vi "Main.vi"() -> ()   [LabVIEW 2017]
doc: "The myRIO Project template acquires acceleration data from the onboard accelerometer and displays the changes of acceleration values in a waveform chart."
uses:
  <vilib>/myRIO/Instrument Drivers/Onboard IO/DIO/typedefs/DIO Reference.ctl
  <vilib>/myRIO/Common/Instrument Driver Framework/Utilities/typedefs/myRIO Generic Hardware Reference.ctl
  <vilib>/myRIO/Common/Instrument Driver Framework/Utilities/typedefs/Hardware Version Enum.ctl
  <vilib>/myRIO/Common/Instrument Driver Framework/Utilities/typedefs/myRIO v1.0 Reference.ctl
  <vilib>/myRIO/Common/Instrument Driver Framework/Utilities/typedefs/Generic FPGA Reference.ctl
  <vilib>/myRIO/Common/Instrument Driver Framework/myRIO v1.0/DIO/typedefs/DIO Channels List.ctl
  <vilib>/myRIO/Common/Instrument Driver Framework/myRIO v1.0/DIO/typedefs/DIO Channels Enum.ctl
  <vilib>/userdefined/High Color/nirio_resource_hc.ctl
  <vilib>/myRIO/Instrument Drivers/Onboard IO/AI/typedefs/AI Reference.ctl
  <vilib>/myRIO/Common/Instrument Driver Framework/myRIO v1.0/AI/typedefs/AI Channels List.ctl
  <vilib>/myRIO/Common/Instrument Driver Framework/myRIO v1.0/AI/typedefs/AI Channels Enum.ctl
  <vilib>/myRIO/Common/Instrument Driver Framework/Utilities/typedefs/Analog Scaling Constants List.ctl
  <vilib>/myRIO/Common/Instrument Driver Framework/Utilities/typedefs/Analog Scaling Constants.ctl
  <vilib>/myRIO/Instrument Drivers/Onboard Devices/Accelerometer/typedefs/Accelerometer Reference.ctl
  <vilib>/myRIO/Common/Instrument Driver Framework/myRIO v1.0/Accelerometer/typedefs/Accelerometer Channels List.ctl
  <vilib>/myRIO/Common/Instrument Driver Framework/myRIO v1.0/Accelerometer/typedefs/Accelerometer Channels Enum.ctl
  <vilib>/myRIO/Instrument Drivers/Onboard IO/PWM/typedefs/PWM Reference.ctl
  <vilib>/myRIO/Common/Instrument Driver Framework/myRIO v1.0/PWM/typedefs/PWM Channels Enum.ctl
  <vilib>/myRIO/Instrument Drivers/Onboard IO/PWM/typedefs/PWM Configuration.ctl
  <vilib>/myRIO/Common/Instrument Driver Framework/Utilities/vis/Is FPGA Ref Available.vi
  <vilib>/myRIO/Common/Instrument Driver Framework/myRIO v1.0/DIO/vis/myRIO v1.1 Open DIO.vi
  <vilib>/myRIO/Instrument Drivers/Onboard IO/DIO/vis/Write.vi
  <vilib>/myRIO/Instrument Drivers/Onboard IO/DIO/vis/Read.vi
  <vilib>/myRIO/Common/Instrument Driver Framework/myRIO v1.0/PWM/vis/myRIO v1.1 Open PWM.vi
  <vilib>/myRIO/Instrument Drivers/Onboard IO/PWM/vis/Set Duty Cycle and Frequency.vi
  <vilib>/myRIO/Common/Instrument Driver Framework/myRIO v1.0/Accelerometer/vis/myRIO v1.1 Open Accelerometer.vi
  <vilib>/myRIO/Instrument Drivers/Onboard Devices/Accelerometer/vis/Read.vi
  <vilib>/myRIO/Common/Instrument Driver Framework/myRIO v1.0/AI/vis/myRIO v1.1 Open AI.vi
  <vilib>/myRIO/Instrument Drivers/Onboard IO/AI/vis/Read.vi
  <vilib>/myRIO/Common/Instrument Driver Framework/Utilities/vis/Validate Channels.vi
  <vilib>/myRIO/Common/Instrument Driver Framework/myRIO v1.0/DIO/vis/myRIO v1.0 Reserve DIO.vi
  <vilib>/myRIO/Common/Instrument Driver Framework/myRIO v1.0/PWM/vis/myRIO v1.0 Reserve PWM.vi
  <vilib>/myRIO/Common/Instrument Driver Framework/myRIO v1.0/Accelerometer/vis/myRIO v1.0 Reserve Accelerometer.vi
  <vilib>/myRIO/Common/Instrument Driver Framework/myRIO v1.0/AI/vis/myRIO v1.0 Reserve AI.vi
  <vilib>/myRIO/Common/Instrument Driver Framework/myRIO v1.0/UART/vis/myRIO v1.0 Close UART.vi
  <vilib>/myRIO/Common/Instrument Driver Framework/myRIO v1.0/Resource Manager/vis/myRIO v1.0 Reserve Channel List.vi
  <vilib>/myRIO/Common/Instrument Driver Framework/myRIO v1.0/DIO/vis/myRIO v1.0 Build MUX Configuration DIO.vi
  <vilib>/myRIO/Common/Instrument Driver Framework/myRIO v1.0/PWM/vis/myRIO v1.0 Build MUX Configuration PWM.vi
  <vilib>/myRIO/Common/Instrument Driver Framework/myRIO v1.0/Accelerometer/vis/myRIO v1.0 Build MUX Configuration Accelerometer.vi
  <vilib>/myRIO/Common/Instrument Driver Framework/myRIO v1.0/AI/vis/myRIO v1.0 Build MUX Configuration AI.vi
  <vilib>/myRIO/Common/Instrument Driver Framework/myRIO v1.0/Resource Manager/vis/myRIO v1.0 Reserve Channel.vi
  <vilib>/myRIO/Common/Instrument Driver Framework/myRIO v1.0/Resource Manager/vis/myRIO v1.0 Unreserve Channel.vi
  <vilib>/myRIO/Common/Instrument Driver Framework/myRIO v1.0/Resource Manager/vis/myRIO v1.0 Create Configuration List.vi
  <vilib>/myRIO/Common/Instrument Driver Framework/myRIO v1.0/Resource Manager/vis/myRIO v1.0 Build Mutex Name.vi
  <vilib>/Utility/VariantDataType/GetNumericInfo.vi
  <vilib>/Utility/error.llb/Error Cluster From Error Code.vi
  <vilib>/myRIO/Common/Instrument Driver Framework/myRIO v1.0/myRIO v1.1 Open.vi
  <vilib>/myRIO/Common/Instrument Driver Framework/Utilities/vis/IO Manager.vi
  <vilib>/myRIO/Common/Instrument Driver Framework/Utilities/vis/Configuration Manager.vi
  <vilib>/myRIO/Common/Instrument Driver Framework/myRIO v1.0/Resource Manager/vis/myRIO v1.0 Configure IO.vi
  <vilib>/myRIO/Common/Instrument Driver Framework/myRIO v1.0/myRIO v1.0 Close.vi
  <vilib>/myRIO/Common/Instrument Driver Framework/myRIO v1.0/DIO/vis/myRIO v1.0 Write DIO.vi
  <vilib>/myRIO/Common/Instrument Driver Framework/myRIO v1.0/AI/vis/myRIO v1.0 Get Scaling Constants AI.vi
  <vilib>/myRIO/Common/Instrument Driver Framework/myRIO v1.0/AI/vis/myRIO v1.0 Read AI.vi
  <vilib>/myRIO/Common/Instrument Driver Framework/myRIO v1.0/Accelerometer/vis/myRIO v1.0 Get Scaling Constant Accelerometer.vi
  <vilib>/myRIO/Common/Instrument Driver Framework/myRIO v1.0/Accelerometer/vis/myRIO v1.0 Read Accelerometer.vi
  <vilib>/myRIO/Common/Instrument Driver Framework/myRIO v1.0/DIO/vis/myRIO v1.0 Read DIO.vi
  <vilib>/myRIO/Common/Instrument Driver Framework/myRIO v1.0/PWM/vis/myRIO v1.0 Write PWM.vi
  <vilib>/myRIO/Common/Instrument Driver Framework/Utilities/vis/FPGA Ref Manager.vi
  <vilib>/myRIO/Common/Instrument Driver Framework/myRIO v1.0/myRIO v1.0 Reset FPGA.vi
  <vilib>/myRIO/Common/Instrument Driver Framework/myRIO v1.0/IRQ/vis/myRIO v1.0 IRQ Info FGV.vi
  <vilib>/myRIO/Common/Instrument Driver Framework/myRIO v1.0/IRQ/vis/myRIO v1.0 Timer IRQ Info FGV.vi
  <vilib>/myRIO/Common/Instrument Driver Framework/myRIO v1.0/IRQ/vis/myRIO v1.0 ISR Agent.vi
  <vilib>/myRIO/Express VI/Onboard Devices/LED/LED Express VI.xnode
  <vilib>/myRIO/Instrument Drivers/Onboard IO/DIO/vis/myRIO DIO Open.xnode
  <vilib>/myRIO/Express VI/Onboard IO/AI/AI Express VI.xnode
  <vilib>/myRIO/Instrument Drivers/Onboard IO/AI/vis/myRIO AI Open.xnode
  <vilib>/myRIO/Express VI/Onboard Devices/Accelerometer/Accelerometer Express VI.xnode
  <vilib>/myRIO/Instrument Drivers/Onboard Devices/Accelerometer/vis/myRIO Accelerometer Open.xnode
  <vilib>/myRIO/Express VI/Onboard Devices/Button/Button Express VI.xnode
  <vilib>/myRIO/Express VI/Onboard IO/PWM/PWM Express VI.xnode
  <vilib>/myRIO/Instrument Drivers/Onboard IO/PWM/vis/myRIO PWM Open.xnode
  <vilib>/myRIO/Instrument Drivers/Utilities/Utilities.lvlib
  <vilib>/myRIO/Instrument Drivers/Onboard IO/AI/AI.lvlib
  <vilib>/myRIO/Instrument Drivers/Onboard IO/PWM/PWM.lvlib
  <vilib>/myRIO/Instrument Drivers/Onboard IO/DIO/DIO.lvlib
  <vilib>/myRIO/Instrument Drivers/Onboard Devices/Accelerometer/Accelerometer.lvlib
panel:
  out "Valve Open":bool
  out "TCP Listen":bool
  out "Reset":bool
  out "Z-Axis":dbl
  out "Y-Axis":dbl
  out "X-Axis":dbl
  out "Accelerometer":cluster{dbl, dbl, dbl}(graph)
  out "Temperature\nMeter":dbl(knob) scale=0.0..100.0
  in  "Max Temperature":dbl
  in  "Front Controller Password":dbl
  in  "STOP SYSTEM":bool
  in  "Max Movement":dbl min=1.0
  out "Self-destruct Timer":i32
  out "Mode":string
  out "Self-destruct Cancelled":bool
  out "Local Cooling Request":bool
  out "Self-destructed":bool
  out "Self-destruct Timer":bool
  out "Movement Detected":bool
  out "Instructions":string
  out "Message Number":dbl
  out "Received Cluster":T1
  out "Front Controller":bool
  out "Local":bool
  out "Bytes written":i32
  out "Send Cluster":T2
  # "LED Indicators"
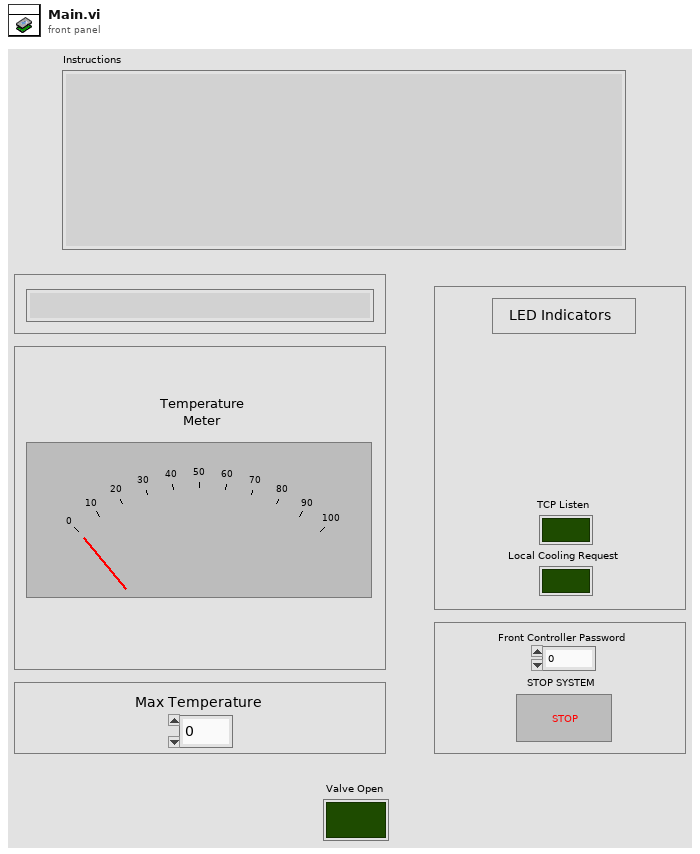
[diagram p1: front panel]
types:
  T1 = cluster{"Servo Open":bool, "Self-Destruct":bool, "Front Controller Passcode":dbl}
  T2 = cluster{"Temperature":dbl, "X - Axis":dbl, "Y - Axis":dbl, "Z - Axis":dbl, "Movement":bool, "Message":dbl, "LCR":bool, "Numeric":dbl}
  T3 = typedef "DIO.lvlib/DIO Reference.ctl" = cluster{"myRIO Reference":T4, "DIO Channels List":T8}
  T4 = typedef "myRIO Generic Hardware Reference.ctl" = cluster{"myRIO Model":T5, "myRIO Hardware Reference":T6}
  T5 = typedef "Hardware Version Enum.ctl" = enum16{"Unknown", "myRIO-1900", "myRIO-1950", "roboRIO", "NI ELVIS RIO CM"}
  T6 = typedef "myRIO v1.0 Reference.ctl" = cluster{"Generic FPGA Reference":T7, "Allow multiple opens":bool}
  T7 = typedef "Generic FPGA Reference.ctl" = refnum<k20>
  T8 = typedef "DIO Channels List.ctl" = T9[]
  T9 = typedef "DIO Channels Enum.ctl" = enum16{"Not Connected", "C/DIO0", "C/DIO1", "C/DIO2", "C/DIO3", "C/DIO4", "C/DIO5", "C/DIO6", "C/DIO7", "A/DIO0", "A/DIO1", "A/DIO2", "A/DIO3", "A/DIO4", "A/DIO5", "A/DIO6", "A/DIO7", "A/DIO8", "A/DIO9", "A/DIO10", "A/DIO11", "A/DIO12", "A/DIO13", "A/DIO14", "A/DIO15", "B/DIO0", "B/DIO1", "B/DIO2", "B/DIO3", "B/DIO4", "B/DIO5", "B/DIO6", "B/DIO7", "B/DIO8", "B/DIO9", "B/DIO10", "B/DIO11", "B/DIO12", "B/DIO13", "B/DIO14", "B/DIO15", "LED0", "LED1", "LED2", "LED3", "Button0", "DIO/DIO0", "DIO/DIO1", "DIO/DIO2", "DIO/DIO3", "DIO/DIO4", "DIO/DIO5", "DIO/DIO6", "DIO/DIO7", "DIO/DIO8", "DIO/DIO9", "SPI/CS0", "SPI/CS1", "SPI/CS2", "SPI/CS3", "LED RADIO (Green)", "LED RADIO (Red)", "LED COMM (Green)", "LED COMM (Red)", "LED MODE (Green)", "LED MODE (Red)"}
  T10 = typedef "nirio_resource_hc.ctl" = tag
  T11 = typedef "PWM.lvlib/PWM Reference.ctl" = cluster{"myRIO Reference":T4, "PWM Channels Enum":T12, "PWM Configuration":T13}
  T12 = typedef "PWM Channels Enum.ctl" = enum16{"Not Connected", "C/PWM0", "C/PWM1", "A/PWM0", "A/PWM1", "A/PWM2", "B/PWM0", "B/PWM1", "B/PWM2", "PWM/PWM0", "PWM/PWM1", "PWM/PWM2", "PWM/PWM3", "PWM/PWM4", "PWM/PWM5", "PWM/PWM6", "PWM/PWM7", "PWM/PWM8", "PWM/PWM9"}
  T13 = typedef "PWM.lvlib/PWM Configuration.ctl" = cluster{"Frequency":dbl, "Duty Cycle":dbl}
  T14 = typedef "Accelerometer.lvlib/Accelerometer Reference.ctl" = cluster{"myRIO Reference":T4, "Accelerometer Channels List":T15, "LSB Weight":dbl}
  T15 = typedef "Accelerometer Channels List.ctl" = T16[]
  T16 = typedef "Accelerometer Channels Enum.ctl" = enum16{"Not Connected", "X-Axis", "Y-Axis", "Z-Axis"}
  T17 = typedef "AI.lvlib/AI Reference.ctl" = cluster{"myRIO Reference":T4, "AI Channels List":T18, "AI Scaling Constants List":T20}
  T18 = typedef "AI Channels List.ctl" = T19[]
  T19 = typedef "AI Channels Enum.ctl" = enum16{"Not Connected", "AudioIn/Left", "AudioIn/Right", "C/AI0", "C/AI1", "A/AI0", "A/AI1", "A/AI2", "A/AI3", "B/AI0", "B/AI1", "B/AI2", "B/AI3", "AI/AI0", "AI/AI1", "AI/AI2", "AI/AI3"}
  T20 = typedef "Analog Scaling Constants List.ctl" = T21[]
  T21 = typedef "Analog Scaling Constants.ctl" = cluster{"LSB Weight (Volts)":dbl, "Offset (Volts)":dbl, "Signed?":bool}
  T22 = cluster{dbl, "X-Axis":dbl, "Y-Axis":dbl, dbl, "Movement Detected":bool, "Message Number":dbl, "Local Cooling Request":bool, "Front Controller Password":dbl}
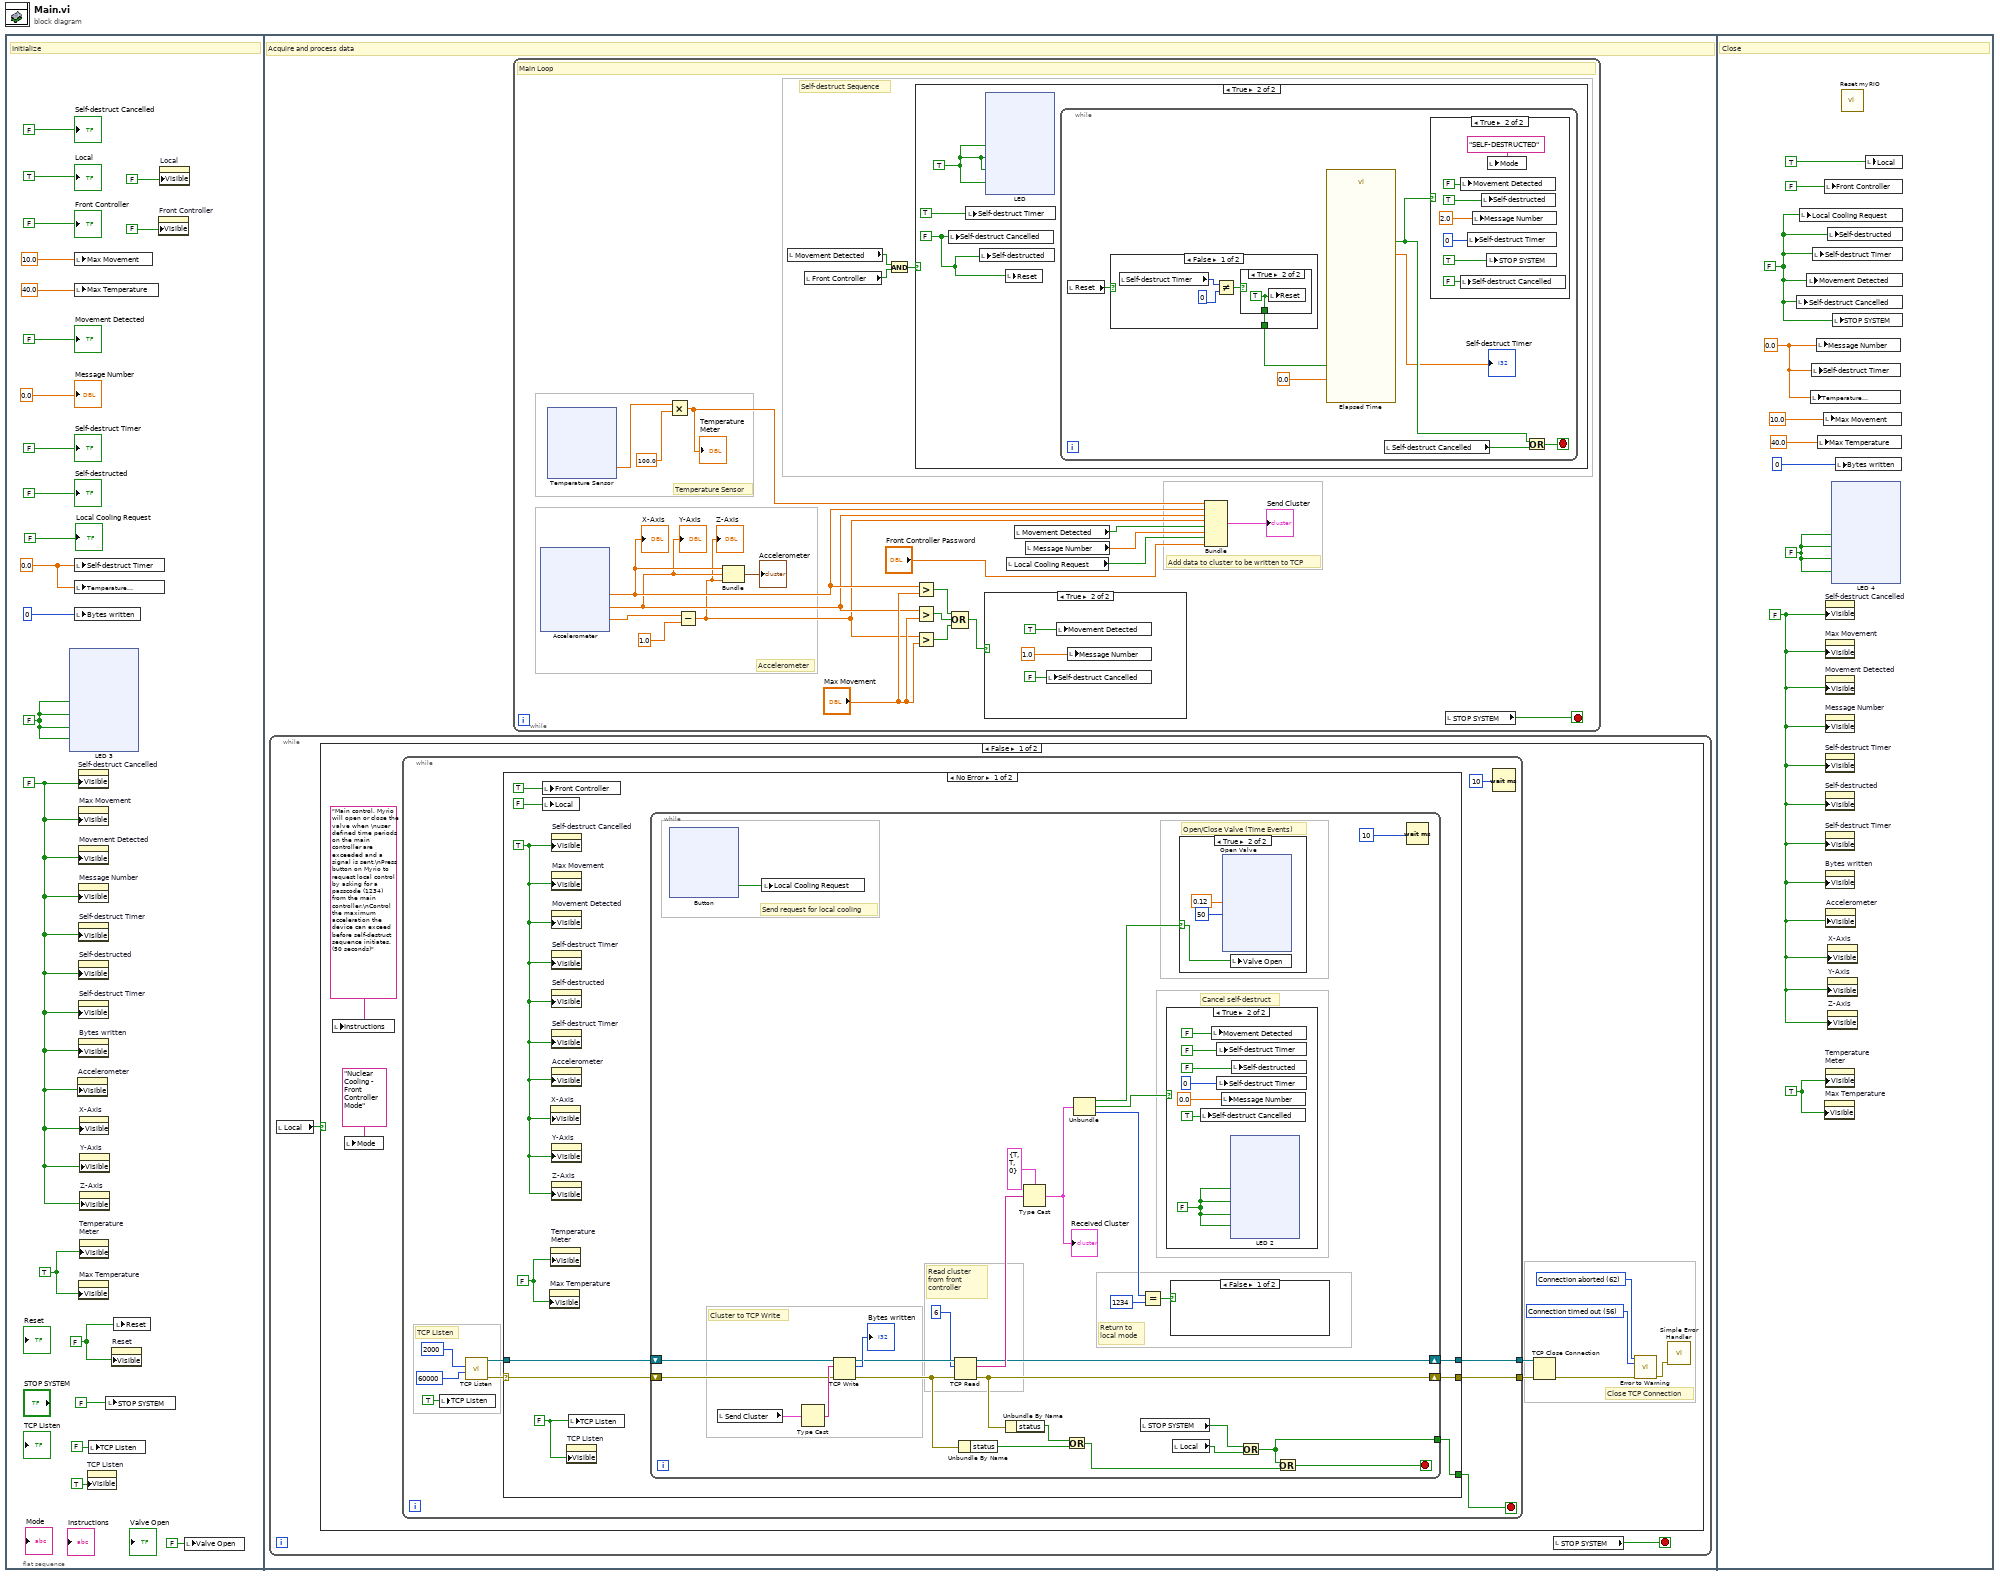
[diagram p0: block diagram]
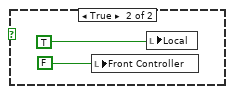
[diagram p2: hidden frame]
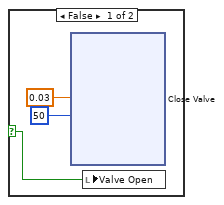
[diagram p4: hidden frame]
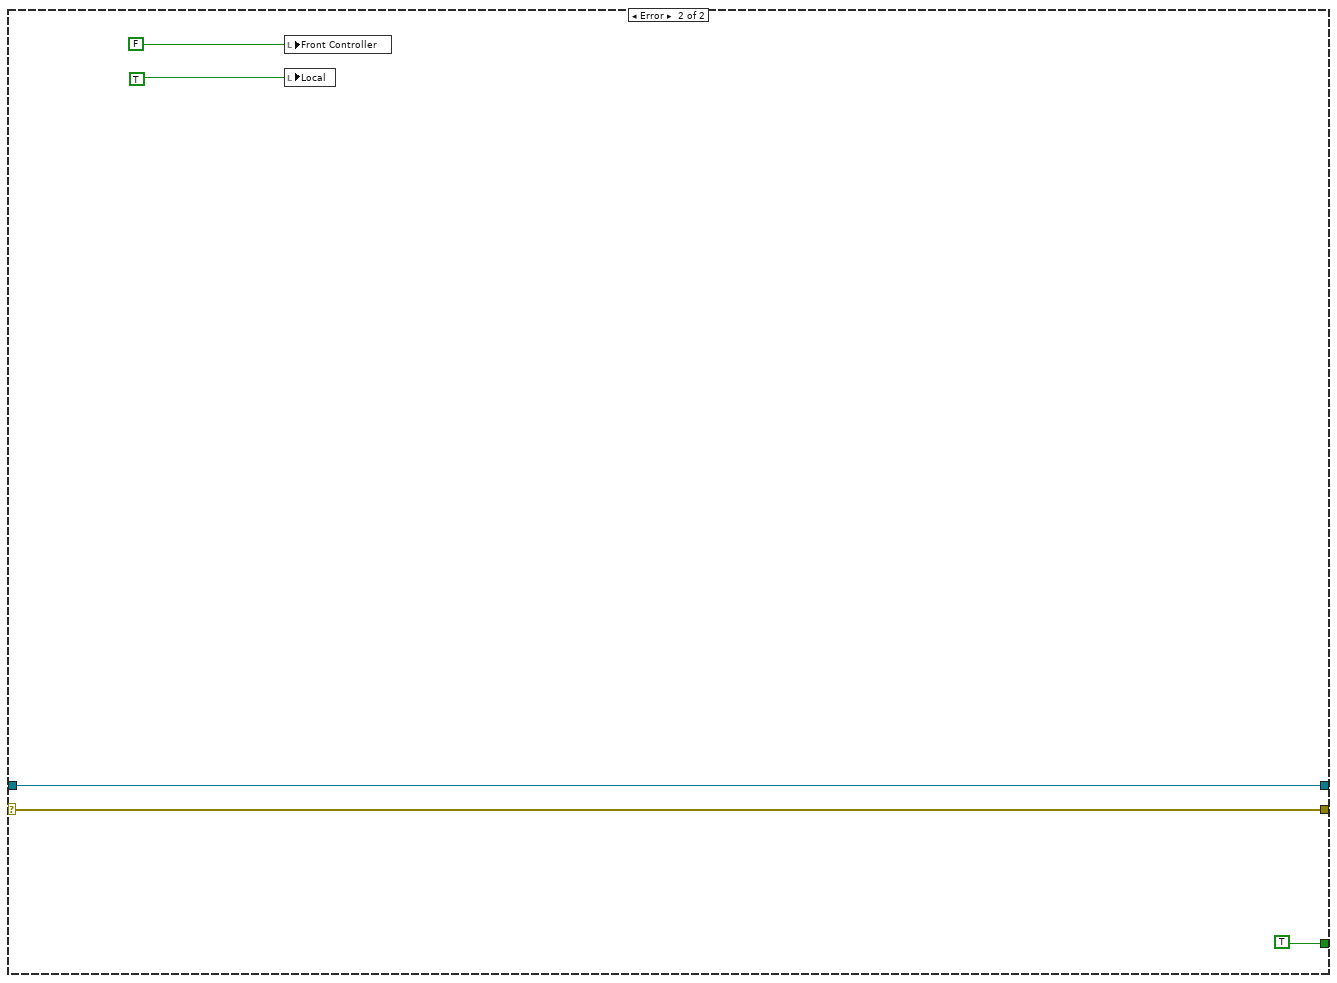
[diagram p5: hidden frame]
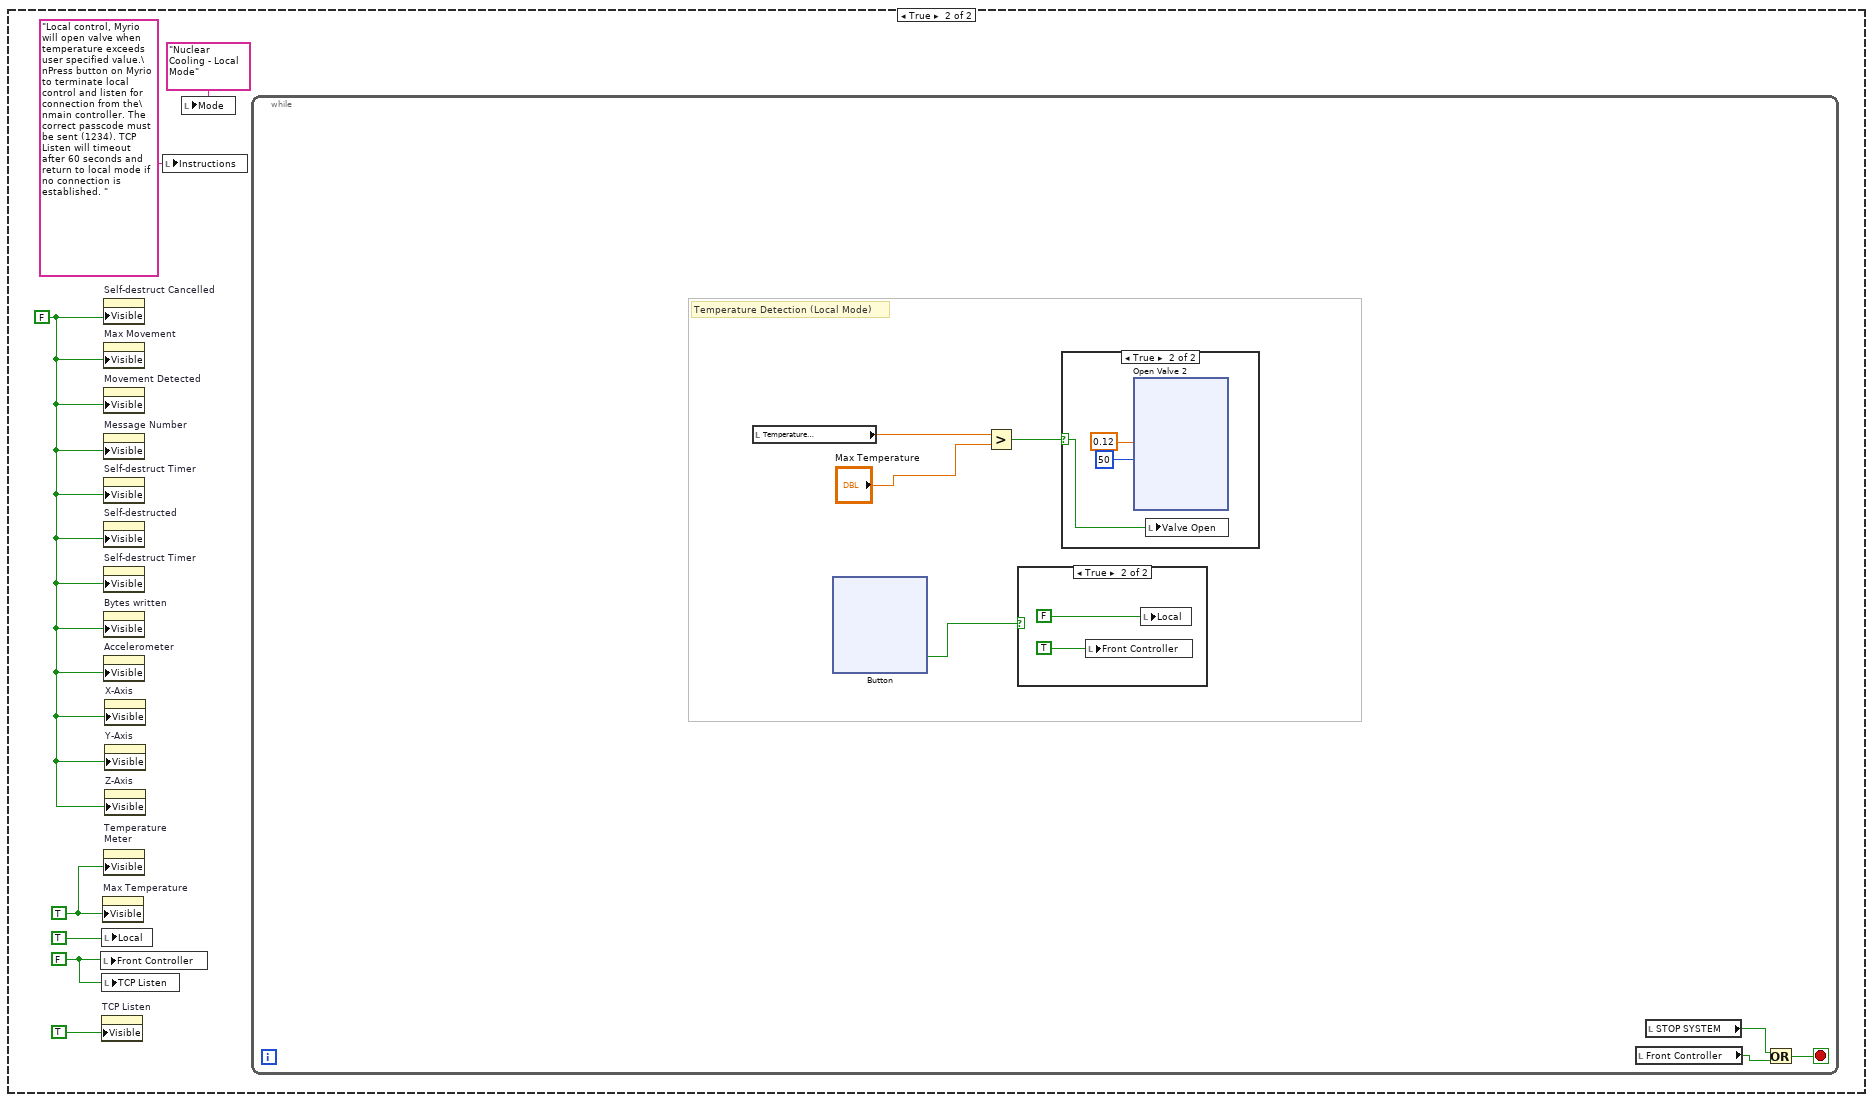
[diagram p6: hidden frame]
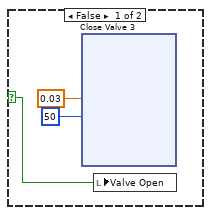
[diagram p8: hidden frame]
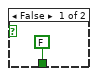
[diagram p10: hidden frame]
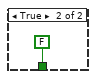
[diagram p11: hidden frame]
diagram:
  n1 = flat-sequence {
    frame #0 {
      w2 = FALSE
      w6 = TRUE
      w5 = FALSE
      w15 = FALSE
      w7 = 0.0
      # "Initialize"
      n2 = xnode "LED 3"("LED0"=w15, "LED1"=w15, "LED2"=w15, "LED3"=w15) -> ()  [unwired: 1 in, 1 out]
      n3 = local write "Max Movement"(10.0) -> ()
      n4 = local write "Max Temperature"(40.0) -> ()
      n5 = local write "Self-destruct Timer"(w7) -> ()
      n6 = local write "Temperature\nMeter"(w7) -> ()
      n7 = local write "Bytes written"(0) -> ()
      n8 = property on="Accelerometer" class="WFChart (strict)"("Visible"=w5) -> ()  [unwired: 2 in, 2 out]
      n9 = property on="Self-destruct Cancelled" class="Bool (strict)"("Visible"=w5) -> ()  [unwired: 2 in, 2 out]
      n10 = property on="Max Movement" class="DigNum (strict)"("Visible"=w5) -> ()  [unwired: 2 in, 2 out]
      n11 = property on="Movement Detected" class="Bool (strict)"("Visible"=w5) -> ()  [unwired: 2 in, 2 out]
      n12 = property on="Message Number" class="DigNum (strict)"("Visible"=w5) -> ()  [unwired: 2 in, 2 out]
      n13 = property on="Self-destruct Timer" class="Bool (strict)"("Visible"=w5) -> ()  [unwired: 2 in, 2 out]
      n14 = property on="Self-destructed" class="Bool (strict)"("Visible"=w5) -> ()  [unwired: 2 in, 2 out]
      n15 = property on="Self-destruct Timer" class="DigNum (strict)"("Visible"=w5) -> ()  [unwired: 2 in, 2 out]
      n16 = property on="Bytes written" class="DigNum (strict)"("Visible"=w5) -> ()  [unwired: 2 in, 2 out]
      n17 = property on="Max Temperature" class="DigNum (strict)"("Visible"=w6) -> ()  [unwired: 2 in, 2 out]
      n18 = property on="X-Axis" class="DigNum (strict)"("Visible"=w5) -> ()  [unwired: 2 in, 2 out]
      n19 = property on="Temperature\nMeter" class="Knob (strict)"("Visible"=w6) -> ()  [unwired: 2 in, 2 out]
      n20 = property on="Y-Axis" class="DigNum (strict)"("Visible"=w5) -> ()  [unwired: 2 in, 2 out]
      n21 = property on="Z-Axis" class="DigNum (strict)"("Visible"=w5) -> ()  [unwired: 2 in, 2 out]
      n22 = property on="TCP Listen" class="Bool (strict)"("Visible"=TRUE) -> ()  [unwired: 2 in, 2 out]
      n23 = local write "TCP Listen"(FALSE) -> ()
      n24 = local write "STOP SYSTEM"(FALSE) -> ()
      n25 = property on="Reset" class="Bool (strict)"("Visible"=w2) -> ()  [unwired: 2 in, 2 out]
      n26 = local write "Reset"(w2) -> ()
      n27 = property on="Front Controller" class="Bool (strict)"("Visible"=FALSE) -> ()  [unwired: 2 in, 2 out]
      n28 = property on="Local" class="Bool (strict)"("Visible"=FALSE) -> ()  [unwired: 2 in, 2 out]
      n29 = local write "Valve Open"(FALSE) -> ()
      "Local" <- TRUE
      "Front Controller" <- FALSE
      "Movement Detected" <- FALSE
      "Message Number" <- 0.0
      "Self-destruct Timer" <- FALSE
      "Self-destruct Cancelled" <- FALSE
      "Self-destructed" <- FALSE
      "Local Cooling Request" <- FALSE
    }
    frame #1 {
      # "Acquire and process data"
      n30 = while {
        stop <- w61 stop-if-true
        n31 = local read "Local"() -> (w62:bool)
        n32 = case shown="False" w62 {
          frame False {
            w66 = 56 items=["No Error", "Argument Error", "Memory Full", "Out of Zone", "End of File", "File Already Open", "Generic File IO Error", "File Not Found", "File Permission Error", "Disk Full", "Duplicate Path", "Too Many Files Open", "Not Enabled", "Resource File Not Found", "Cannot Add Resource", "Resource Not Found", "Image Not Found", "Image Memory Error", "Pen Does Not Exist", "Config Bad Type", "Config Token Not Found", "Config Parse Error", "Config Memory Error", "Bad External Code Format", "Bad External Code Offset", "External Code Not Present", "Null Window", "Destroy Window Mixup", "Null Menu", "Print Aborted", "Bad Print Record", "Print Driver Error", "Windows Error During Print", "Memory Error During Print", "Print Dialog Error", "Generic Print Error", "Invalid Device Refnum", "Device Not Found", "Device Parameter Error", "Device Unit Error", "Can't Open Device", "Device Call Aborted", "Generic Error", "Cancelled By User", "Object ID Too Low", "Object ID Too High", "Object Not In Heap", "Unknown Heap", "Bad DefProc ID", "DefProc Not In Table", "Message Out Of Range", "Null Method", "Unknown Message", "Manager Call Not Supported", "Bad address", "Connection In progress", "Connection timed out", "Connection is already in progress", "Network attribute not supported", "Network error", "Address in use", "System out of memory", "Connection aborted", "Connection refused", "Connection is not connected", "Connection is already connected", "Connection closed", "Initialize error (interapplication manager)", "Bad occurrence", "Wait on unbound occurrence handler", "Occurrence queue overflow", "Bad path", "Semaphore not signaled", "Unrecognized type (interapplication manager)"] ("3rd Error to Convert")
            w67 = 62 items=["No Error", "Argument Error", "Memory Full", "Out of Zone", "End of File", "File Already Open", "Generic File IO Error", "File Not Found", "File Permission Error", "Disk Full", "Duplicate Path", "Too Many Files Open", "Not Enabled", "Resource File Not Found", "Cannot Add Resource", "Resource Not Found", "Image Not Found", "Image Memory Error", "Pen Does Not Exist", "Config Bad Type", "Config Token Not Found", "Config Parse Error", "Config Memory Error", "Bad External Code Format", "Bad External Code Offset", "External Code Not Present", "Null Window", "Destroy Window Mixup", "Null Menu", "Print Aborted", "Bad Print Record", "Print Driver Error", "Windows Error During Print", "Memory Error During Print", "Print Dialog Error", "Generic Print Error", "Invalid Device Refnum", "Device Not Found", "Device Parameter Error", "Device Unit Error", "Can't Open Device", "Device Call Aborted", "Generic Error", "Cancelled By User", "Object ID Too Low", "Object ID Too High", "Object Not In Heap", "Unknown Heap", "Bad DefProc ID", "DefProc Not In Table", "Message Out Of Range", "Null Method", "Unknown Message", "Manager Call Not Supported", "Bad address", "Connection In progress", "Connection timed out", "Connection is already in progress", "Network attribute not supported", "Network error", "Address in use", "System out of memory", "Connection aborted", "Connection refused", "Connection is not connected", "Connection is already connected", "Connection closed", "Initialize error (interapplication manager)", "Bad occurrence", "Wait on unbound occurrence handler", "Occurrence queue overflow", "Bad path", "Semaphore not signaled", "Unrecognized type (interapplication manager)"] ("1st Error to Convert")
            # "Close TCP Connection"
            n33 = local write "Instructions"("Main control, Myrio will open or close the valve when \nuser defined time periods on the main controller are exceeded and a signal is sent.\nPress button on Myrio to request local control by asking for a passcode (1234) from the main controller.\nControl the maximum acceleration the device can exceed before self-destruct sequence initiates. (50 seconds)") -> ()
            n34 = local write "Mode"("Nuclear Cooling - Front Controller Mode") -> ()
            n35 = while {
              tunnel: [w73] -> w69
              tunnel: [w72] -> w68
              stop <- w76 stop-if-true
              # "TCP Listen"
              n36 = local write "TCP Listen"(TRUE) -> ()
              n37 = call <vilib>:"TCP Listen.vi"("timeout ms (wait forever: -1)"=60000, "port"=u16 2000 ("timeout ms (wait forever: -1)")) -> ("error out"=w75:errorcluster, "connection ID"=w74:refnum<k5>)  [unwired: 2 in, 6 out]
              n38 = case shown="No Error" w75 {
                selector: w75 -> [w89 w278]
                tunnel: [w88 TRUE] -> w76
                tunnel: w74 -> [w87 w279]
                tunnel: [w86 w279] -> w73
                tunnel: [w85 w278] -> w72
                frame No Error {
                  w80 = FALSE
                  w82 = FALSE
                  w81 = TRUE
                  n39 = local write "Front Controller"(TRUE) -> ()
                  n40 = local write "Local"(FALSE) -> ()
                  n41 = property on="Max Temperature" class="DigNum (strict)"("Visible"=w82) -> ()  [unwired: 2 in, 2 out]
                  n42 = property on="X-Axis" class="DigNum (strict)"("Visible"=w81) -> ()  [unwired: 2 in, 2 out]
                  n43 = property on="Temperature\nMeter" class="Knob (strict)"("Visible"=w82) -> ()  [unwired: 2 in, 2 out]
                  n44 = property on="Self-destruct Cancelled" class="Bool (strict)"("Visible"=w81) -> ()  [unwired: 2 in, 2 out]
                  n45 = property on="Max Movement" class="DigNum (strict)"("Visible"=w81) -> ()  [unwired: 2 in, 2 out]
                  n46 = property on="Movement Detected" class="Bool (strict)"("Visible"=w81) -> ()  [unwired: 2 in, 2 out]
                  n47 = property on="Self-destruct Timer" class="Bool (strict)"("Visible"=w81) -> ()  [unwired: 2 in, 2 out]
                  n48 = property on="Self-destructed" class="Bool (strict)"("Visible"=w81) -> ()  [unwired: 2 in, 2 out]
                  n49 = property on="Self-destruct Timer" class="DigNum (strict)"("Visible"=w81) -> ()  [unwired: 2 in, 2 out]
                  n50 = property on="Accelerometer" class="WFChart (strict)"("Visible"=w81) -> ()  [unwired: 2 in, 2 out]
                  n51 = property on="Y-Axis" class="DigNum (strict)"("Visible"=w81) -> ()  [unwired: 2 in, 2 out]
                  n52 = property on="Z-Axis" class="DigNum (strict)"("Visible"=w81) -> ()  [unwired: 2 in, 2 out]
                  n53 = property on="TCP Listen" class="Bool (strict)"("Visible"=w80) -> ()  [unwired: 2 in, 2 out]
                  n54 = local write "TCP Listen"(w80) -> ()
                  n55 = while {
                    shift-right: [w103] -> w86
                    shift-left: w87 -> [w112]
                    shift-right: [w102] -> w85
                    shift-left: w89 -> [w114]
                    tunnel: [w90] -> w88
                    stop <- w104 stop-if-true
                    # "Return to \nlocal mode"
                    # "Cancel self-destruct"
                    # "Open/Close Valve (Time Events)"
                    # "Read cluster \nfrom front controller"
                    # "Send request for local cooling"
                    # "Cluster to TCP Write"
                    n56 = xnode "Button"() -> ("Value"=w96:bool)  [unwired: 1 in, 1 out]
                    n57 = local read "Send Cluster"() -> (w113:T2)
                    n58 = local write "Local Cooling Request"(w96) -> ()
                    n59 = Type Cast(x=w113) -> (*(type *) &x=w116:string)  [unwired: 1 out]
                    n60 = TCP Write(connection ID=w112, data in=w116, error in (no error)=w114) -> (connection ID out=w111:refnum<k5>, bytes written=→"Bytes written":i32, error out=w108:errorcluster)  [unwired: 1 out]
                    n61 = TCP Read(connection ID=w111, bytes to read=6, error in (no error)=w108) -> (connection ID out=w103:refnum<k5>, data out=w109:string, error out=w102:errorcluster)  [unwired: 2 in]
                    n62 = Unbundle By Name(w108) -> ("status"=w107:bool)
                    n63 = Unbundle By Name(w102) -> ("status"=w106:bool)
                    n64 = Type Cast(type=cluster{bool, bool, i32} {TRUE, TRUE, 0}, x=w109) -> (*(type *) &x=w100:cluster{bool, bool, i32})
                    "Received Cluster" <- w100
                    n65 = Or(x=w106, y=w107) -> (x .or. y?=w105:bool)
                    n66 = Unbundle(w100) -> (w97:bool, w98:bool, w93:i32)
                    n67 = local read "STOP SYSTEM"() -> (w92:bool)
                    n68 = Equal?(x=w93, y=1234) -> (x = y?=w95:bool)
                    n69 = case shown="True" w98 {
                      frame False {
                      }
                      frame True {
                        w155 = FALSE
                        n70 = local write "Self-destruct Cancelled"(TRUE) -> ()
                        n71 = local write "Movement Detected"(FALSE) -> ()
                        n72 = local write "Self-destruct Timer"(FALSE) -> ()
                        n73 = local write "Self-destruct Timer"(0) -> ()
                        n74 = local write "Message Number"(0.0) -> ()
                        n75 = xnode "LED 2"("LED0"=w155, "LED1"=w155, "LED2"=w155, "LED3"=w155) -> ()  [unwired: 1 in, 1 out]
                        n76 = local write "Self-destructed"(FALSE) -> ()
                      }
                    }
                    n77 = case shown="False" w95 {
                      frame False {
                      }
                      frame True {
                        n78 = local write "Front Controller"(FALSE) -> ()
                        n79 = local write "Local"(TRUE) -> ()
                      }
                    }
                    n80 = local read "Local"() -> (w91:bool)
                    n81 = case shown="True" w97 {
                      selector: w97 -> [w199 w237]
                      frame False {
                        n82 = xnode "Close Valve"("Duty Cycle"=0.03, "Frequency [Hz]"=50) -> ()  [unwired: 1 in, 1 out]
                        n83 = local write "Valve Open"(w199) -> ()
                      }
                      frame True {
                        n84 = xnode "Open Valve"("Duty Cycle"=0.12, "Frequency [Hz]"=50) -> ()  [unwired: 1 in, 1 out]
                        n85 = local write "Valve Open"(w237) -> ()
                      }
                    }
                    n86 = Or(x=w92, y=w91) -> (x .or. y?=w90:bool)
                    n87 = Or(x=w90, y=w105) -> (x .or. y?=w104:bool)
                    n88 = Wait (ms)(milliseconds to wait=u32 10) -> ()  [unwired: 1 out]
                  }
                }
                frame Error {
                  n89 = local write "Front Controller"(FALSE) -> ()
                  n90 = local write "Local"(TRUE) -> ()
                }
              }
              n91 = Wait (ms)(milliseconds to wait=u32 10) -> ()  [unwired: 1 out]
            }
            n92 = TCP Close Connection(connection ID=w69, error in (no error)=w68) -> (error out=w65:errorcluster)  [unwired: 2 out]
            n93 = call <vilib>:"Error to Warning.vi"("1st Error to Convert"=w67, "2nd Error to Convert"=w66, "error in"=w65) -> ("warning out"=w64:errorcluster)  [unwired: 3 in, 9 out]
            n94 = call <vilib>:"Simple Error Handler.vi"("error in (no error)"=w64) -> ()  [unwired: 1 in, 8 out]
          }
          frame True {
            w282 = FALSE
            w284 = TRUE
            w283 = FALSE
            n95 = local write "Front Controller"(w282) -> ()
            n96 = local write "Local"(TRUE) -> ()
            n97 = local write "TCP Listen"(w282) -> ()
            n98 = property on="TCP Listen" class="Bool (strict)"("Visible"=TRUE) -> ()  [unwired: 2 in, 2 out]
            n99 = property on="Max Temperature" class="DigNum (strict)"("Visible"=w284) -> ()  [unwired: 2 in, 2 out]
            n100 = property on="Self-destruct Cancelled" class="Bool (strict)"("Visible"=w283) -> ()  [unwired: 2 in, 2 out]
            n101 = property on="Max Movement" class="DigNum (strict)"("Visible"=w283) -> ()  [unwired: 2 in, 2 out]
            n102 = property on="Movement Detected" class="Bool (strict)"("Visible"=w283) -> ()  [unwired: 2 in, 2 out]
            n103 = property on="Message Number" class="DigNum (strict)"("Visible"=w283) -> ()  [unwired: 2 in, 2 out]
            n104 = property on="Self-destruct Timer" class="Bool (strict)"("Visible"=w283) -> ()  [unwired: 2 in, 2 out]
            n105 = property on="Self-destructed" class="Bool (strict)"("Visible"=w283) -> ()  [unwired: 2 in, 2 out]
            n106 = property on="Self-destruct Timer" class="DigNum (strict)"("Visible"=w283) -> ()  [unwired: 2 in, 2 out]
            n107 = property on="Bytes written" class="DigNum (strict)"("Visible"=w283) -> ()  [unwired: 2 in, 2 out]
            n108 = property on="Accelerometer" class="WFChart (strict)"("Visible"=w283) -> ()  [unwired: 2 in, 2 out]
            n109 = property on="Temperature\nMeter" class="Knob (strict)"("Visible"=w284) -> ()  [unwired: 2 in, 2 out]
            n110 = property on="X-Axis" class="DigNum (strict)"("Visible"=w283) -> ()  [unwired: 2 in, 2 out]
            n111 = property on="Y-Axis" class="DigNum (strict)"("Visible"=w283) -> ()  [unwired: 2 in, 2 out]
            n112 = property on="Z-Axis" class="DigNum (strict)"("Visible"=w283) -> ()  [unwired: 2 in, 2 out]
            n113 = local write "Instructions"("Local control, Myrio will open valve when temperature exceeds user specified value.\nPress button on Myrio to terminate local control and listen for connection from the\nmain controller. The correct passcode must be sent (1234). TCP Listen will timeout after 60 seconds and return to local mode if no connection is established. ") -> ()
            n114 = local write "Mode"("Nuclear Cooling - Local Mode") -> ()
            n115 = while {
              stop <- w290 stop-if-true
              # "Temperature Detection (Local Mode)"
              n116 = local read "Temperature\nMeter"() -> (w287:dbl)
              n117 = xnode "Button"() -> ("Value"=w292:bool)  [unwired: 1 in, 1 out]
              n118 = Greater?(x=w287, y="Max Temperature") -> (0:w293:bool)
              n119 = case shown="True" w292 {
                frame False {
                }
                frame True {
                  n120 = local write "Front Controller"(TRUE) -> ()
                  n121 = local write "Local"(FALSE) -> ()
                }
              }
              n122 = case shown="True" w293 {
                selector: w293 -> [w331 w369]
                frame False {
                  n123 = xnode "Close Valve 3"("Duty Cycle"=0.03, "Frequency [Hz]"=50) -> ()  [unwired: 1 in, 1 out]
                  n124 = local write "Valve Open"(w331) -> ()
                }
                frame True {
                  n125 = xnode "Open Valve 2"("Duty Cycle"=0.12, "Frequency [Hz]"=50) -> ()  [unwired: 1 in, 1 out]
                  n126 = local write "Valve Open"(w369) -> ()
                }
              }
              n127 = local read "Front Controller"() -> (w289:bool)
              n128 = local read "STOP SYSTEM"() -> (w288:bool)
              n129 = Or(x=w288, y=w289) -> (x .or. y?=w290:bool)
            }
          }
        }
        n130 = local read "STOP SYSTEM"() -> (w61:bool)
      }
      n131 = while {
        stop <- w417 stop-if-true
        # "Self-destruct Sequence"
        # "Add data to cluster to be written to TCP"
        # "Accelerometer"
        # "Temperature Sensor"
        # "Main Loop"
        n132 = xnode "Accelerometer"() -> ("X-Axis"=w409:dbl, "Y-Axis"=w408:dbl, "Z-Axis"=w411:dbl)  [unwired: 1 in, 1 out]
        "X-Axis" <- w409
        "Y-Axis" <- w408
        n133 = xnode "Temperature Sensor"() -> ("A/AI3 (Pin 9)"=w429:dbl)  [unwired: 1 in, 1 out]
        n134 = Multiply(x=w429, y=100.0) -> (x*y=w412:dbl)
        "Temperature\nMeter" <- w412
        n135 = Subtract(x=w411, y=1.0) -> (x-y=w407:dbl)
        "Z-Axis" <- w407
        n136 = Bundle("X-Axis"=w409, "Y-Axis"=w408, w407) -> (→"Accelerometer":cluster{"X-Axis":dbl, "Y-Axis":dbl, dbl})  [unwired: 1 in]
        n137 = local read "Movement Detected"() -> (w413:bool)
        n138 = local read "Front Controller"() -> (w415:bool)
        n139 = And(x=w413, y=w415) -> (x .and. y?=w416:bool)
        n140 = case shown="True" w416 {
          frame False {
          }
          frame True {
            w469 = FALSE
            w470 = TRUE
            n141 = local write "Self-destruct Cancelled"(w469) -> ()
            n142 = local write "Self-destruct Timer"(TRUE) -> ()
            n143 = local write "Self-destructed"(w469) -> ()
            n144 = xnode "LED"("LED0"=w470, "LED1"=w470, "LED2"=w470, "LED3"=w470) -> ()  [unwired: 1 in, 1 out]
            n145 = local write "Reset"(w469) -> ()
            n146 = while {
              stop <- w516 stop-if-true
              n147 = local read "Reset"() -> (w511:bool)
              n148 = case shown="False" w511 {
                tunnel: [w517 FALSE] -> w510
                frame False {
                  n149 = local read "Self-destruct Timer"() -> (w518:i32)
                  n150 = Not Equal?(x=w518, y=0) -> (x != y?=w520:bool)
                  n151 = case shown="True" w520 {
                    tunnel: [FALSE w522] -> w517
                    frame False {
                    }
                    frame True {
                      w522 = TRUE
                      n152 = local write "Reset"(w522) -> ()
                    }
                  }
                }
                frame True {
                }
              }
              n153 = call "Elapsed Time"("Reset"=w510, "Set Start Time (s)"=0.0) -> ("Elapsed Time (s)"=→"Self-destruct Timer":dbl, "Time has Elapsed"=w514:bool)  [unwired: 10 in, 6 out]
              n154 = local read "Self-destruct Cancelled"() -> (w515:bool)
              n155 = case shown="True" w514 {
                frame False {
                }
                frame True {
                  n156 = local write "Self-destruct Cancelled"(FALSE) -> ()
                  n157 = local write "Movement Detected"(FALSE) -> ()
                  n158 = local write "Self-destruct Timer"(0) -> ()
                  n159 = local write "Message Number"(2.0) -> ()
                  n160 = local write "Self-destructed"(TRUE) -> ()
                  n161 = local write "STOP SYSTEM"(TRUE) -> ()
                  n162 = local write "Mode"("SELF-DESTRUCTED") -> ()
                }
              }
              n163 = Or(x=w514, y=w515) -> (x .or. y?=w516:bool)
            }
          }
        }
        n164 = Greater?(x=w409, y="Max Movement") -> (0:w426:bool)
        n165 = Greater?(x=w408, y="Max Movement") -> (0:w425:bool)
        n166 = Greater?(x=w407, y="Max Movement") -> (0:w424:bool)
        n167 = Compound Arithmetic op=OR(w426, w425, w424) -> (w422:bool)
        n168 = case shown="True" w422 {
          frame False {
          }
          frame True {
            n169 = local write "Self-destruct Cancelled"(FALSE) -> ()
            n170 = local write "Movement Detected"(TRUE) -> ()
            n171 = local write "Message Number"(1.0) -> ()
          }
        }
        n172 = local read "Local Cooling Request"() -> (w418:bool)
        n173 = local read "Movement Detected"() -> (w421:bool)
        n174 = local read "Message Number"() -> (w419:dbl)
        n175 = Bundle(w412, "X-Axis"=w409, "Y-Axis"=w408, w407, "Movement Detected"=w421, "Message Number"=w419, "Local Cooling Request"=w418, "Front Controller Password"="Front Controller Password") -> (→"Send Cluster":T22)  [unwired: 1 in]
        n176 = local read "STOP SYSTEM"() -> (w417:bool)
      }
    }
    frame #2 {
      w573 = TRUE
      w571 = FALSE
      w579 = FALSE
      w572 = 0.0
      w575 = FALSE
      # "Close"
      n177 = local write "Self-destruct Cancelled"(w575) -> ()
      n178 = local write "Local Cooling Request"(w575) -> ()
      n179 = local write "Movement Detected"(w575) -> ()
      n180 = local write "Temperature\nMeter"(w572) -> ()
      n181 = local write "Self-destruct Timer"(w572) -> ()
      n182 = local write "Self-destruct Timer"(w575) -> ()
      n183 = local write "Message Number"(w572) -> ()
      n184 = local write "Max Temperature"(40.0) -> ()
      n185 = local write "Max Movement"(10.0) -> ()
      n186 = local write "Front Controller"(FALSE) -> ()
      n187 = property on="Max Temperature" class="DigNum (strict)"("Visible"=w573) -> ()  [unwired: 2 in, 2 out]
      n188 = property on="Self-destruct Cancelled" class="Bool (strict)"("Visible"=w571) -> ()  [unwired: 2 in, 2 out]
      n189 = property on="Max Movement" class="DigNum (strict)"("Visible"=w571) -> ()  [unwired: 2 in, 2 out]
      n190 = property on="Movement Detected" class="Bool (strict)"("Visible"=w571) -> ()  [unwired: 2 in, 2 out]
      n191 = property on="Message Number" class="DigNum (strict)"("Visible"=w571) -> ()  [unwired: 2 in, 2 out]
      n192 = property on="Self-destruct Timer" class="Bool (strict)"("Visible"=w571) -> ()  [unwired: 2 in, 2 out]
      n193 = property on="Self-destructed" class="Bool (strict)"("Visible"=w571) -> ()  [unwired: 2 in, 2 out]
      n194 = property on="Self-destruct Timer" class="DigNum (strict)"("Visible"=w571) -> ()  [unwired: 2 in, 2 out]
      n195 = property on="Bytes written" class="DigNum (strict)"("Visible"=w571) -> ()  [unwired: 2 in, 2 out]
      n196 = property on="Temperature\nMeter" class="Knob (strict)"("Visible"=w573) -> ()  [unwired: 2 in, 2 out]
      n197 = property on="Accelerometer" class="WFChart (strict)"("Visible"=w571) -> ()  [unwired: 2 in, 2 out]
      n198 = local write "Self-destructed"(w575) -> ()
      n199 = property on="X-Axis" class="DigNum (strict)"("Visible"=w571) -> ()  [unwired: 2 in, 2 out]
      n200 = property on="Y-Axis" class="DigNum (strict)"("Visible"=w571) -> ()  [unwired: 2 in, 2 out]
      n201 = property on="Z-Axis" class="DigNum (strict)"("Visible"=w571) -> ()  [unwired: 2 in, 2 out]
      n202 = xnode "LED 4"("LED0"=w579, "LED1"=w579, "LED2"=w579, "LED3"=w579) -> ()  [unwired: 1 in, 1 out]
      n203 = local write "STOP SYSTEM"(w575) -> ()
      n204 = local write "Bytes written"(0) -> ()
      n205 = call <vilib>:"Reset myRIO.vi"() -> ()  [unwired: 11 in, 1 out]
      n206 = local write "Local"(TRUE) -> ()
    }
  }
